vi "IMAQ-MWT DUAL DMD Intensity Calibration (HOST).vi"() -> ()   [LabVIEW 2017]
uses:
  Modules/Common/Controls (HOST)/Image Size.ctl
  Modules/Common/Controls (HOST)/REF.ctl
  Modules/Common/Controls (HOST)/Image Queue Bundle.ctl
  Modules/Common/Controls (HOST)/Data to Disk Bundle.ctl
  Modules/Common/Controls (HOST)/File Name Prefix.ctl
  Modules/Common/Controls (HOST)/FPGA REF (MWT).ctl
  Modules/Common/Controls (HOST)/Main States.ctl
  Modules/Common/Controls (HOST)/IMAQ Parameters.ctl
  Modules/Common/Controls (HOST)/File REF.ctl
  <vilib>/vision/Avi.llb/IMAQ AVI2 Refnum.ctl
  Modules/Common/Controls (HOST)/Experiment Mode.ctl
  <vilib>/Utility/error.llb/Error Cluster From Error Code.vi
  <vilib>/rvi/errors/niLvFpgaAdjustHostInterfaceError.vi
  <vilib>/FPGAPlugInAG/Dynamic/niLvFpga_Close_Dynamic.vi
  <vilib>/Utility/file.llb/Read Delimited Spreadsheet (DBL).vi
  <vilib>/Utility/file.llb/Write Delimited Spreadsheet (DBL).vi
  <vilib>/rvi/interface/nirviReadWriteControl/nirviReadWriteControl.xnode
  <vilib>/rvi/interface/nirviCloseFPGA/nirviCloseFPGA.xnode
  NiFpgaLv.dll
  <vilib>/rvi/interface/Simulation/niFpgaSimulationCallBeginRW.vi
panel:
  in  "Rows Complete":i32
  in  "Int Coeff":bool
  in  "Intensity (mW/cm2)":dbl[][](array[numeric])
  in  "Save Int":bool
  in  "Measured Intensity (uW/cm2)":dbl format="%.2f"
  in  "Current Measurement Spot":cluster{"Rows":u32, "Columns":u32}={"Rows"=1, "Columns"=1} {"Columns" min=1 step=1; "Rows" min=1 step=1}
  out "Total Number of Calibration Points":u32
  in  "Number of Calibration Points":cluster{"Rows":u32, "Columns":u32}={"Rows"=4, "Columns"=4}
  in  "Image Size":T1={"Height"=3072, "Width"=3200}
  out "Frame Rate":u32
  out "Frame #":u32
  in  "Stop Button":bool
  in  "Go":bool
  in  "Height":i32=100
  in  "Width":i32=100
  in  "Y":i32=334
  in  "X":i32=462
  out "Exp. Status":string="Camera Connected"
  out "REF":T2
  out "Command Q":refnum<queue>
  out "Display":T5(plugin-control)
  out "Stopped?":bool
  # "DUAL DMD Intensity Calibration"
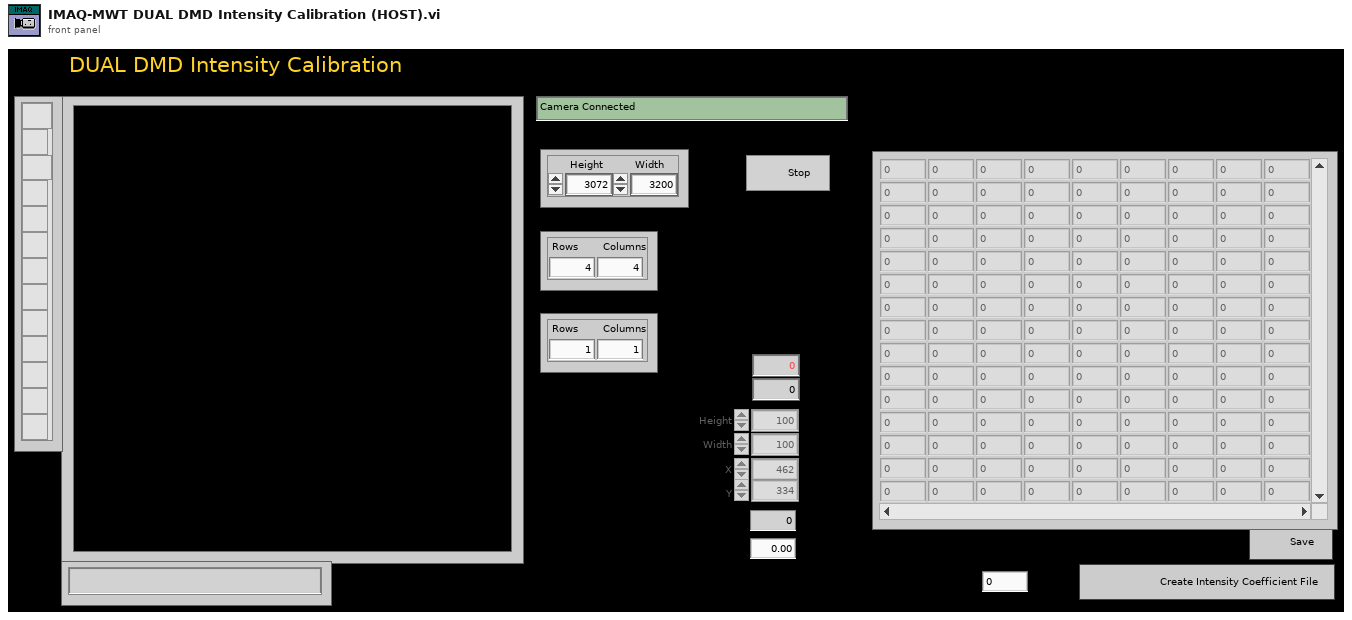
[diagram p1: front panel]
types:
  T1 = typedef "Image Size.ctl" = cluster{"Height":u16, "Width":u16}
  T2 = typedef "REF.ctl" = cluster{"Queue REF":T3, "FPGA REF (MWT)":T4}
  T3 = typedef "Image Queue Bundle.ctl" = cluster{"Disk Image":refnum<queue>, "Image Blocks":refnum<queue>, "Display Image":refnum<queue>, "BG Image":refnum<queue>, "Tag Image":refnum<queue>, "DLL Input":refnum<queue>, "DMD Input":refnum<queue>, "GALVO Input":refnum<queue>}
  T4 = typedef "FPGA REF (MWT).ctl" = refnum<k20>
  T5 = typedef "IMAQ Image.ctl" = refnum<image>
  T6 = enum8{"Enabled", "Disabled", "Disabled and Grayed Out"}
  T7 = typedef "Main States.ctl" = enum16{"Open FPGA", "Initialize", "Preview", "Acquire Images", "STOP"}
  T8 = typedef "Experiment Mode.ctl" = enum16{"Live", "Replay"}
  T9 = typedef "IMAQ Parameters.ctl" = cluster{"File REF":T10, "Frame Data":cluster{"Width":u32, "Height":u32, "Frames Per Second":u32, "Codec":string}, "File Type":string, "Experiment Mode":T8, "Movie File Path":path}
  T10 = typedef "File REF.ctl" = cluster{"AVI REF":T11, "DBDE REF":refnum<file>}
  T11 = typedef "IMAQ AVI2 Refnum.ctl" = refnum<k20>
  T12 = typedef "Data to Disk Bundle.ctl" = cluster{"Frame Number":u64, "Time Stamp (us)":u64, "Image Data":u64[], "Contour":u32[], "Raw Image REF":refnum<data-value>, "Block Image REF":refnum<data-value>, "Block Box":u64[], "SPINE":u32[], "HT Angle":u64[], "Block Position":u64[], "SPINE Count":u32[], "Contour Count":u32[], "SPINE DIR":u8[]}
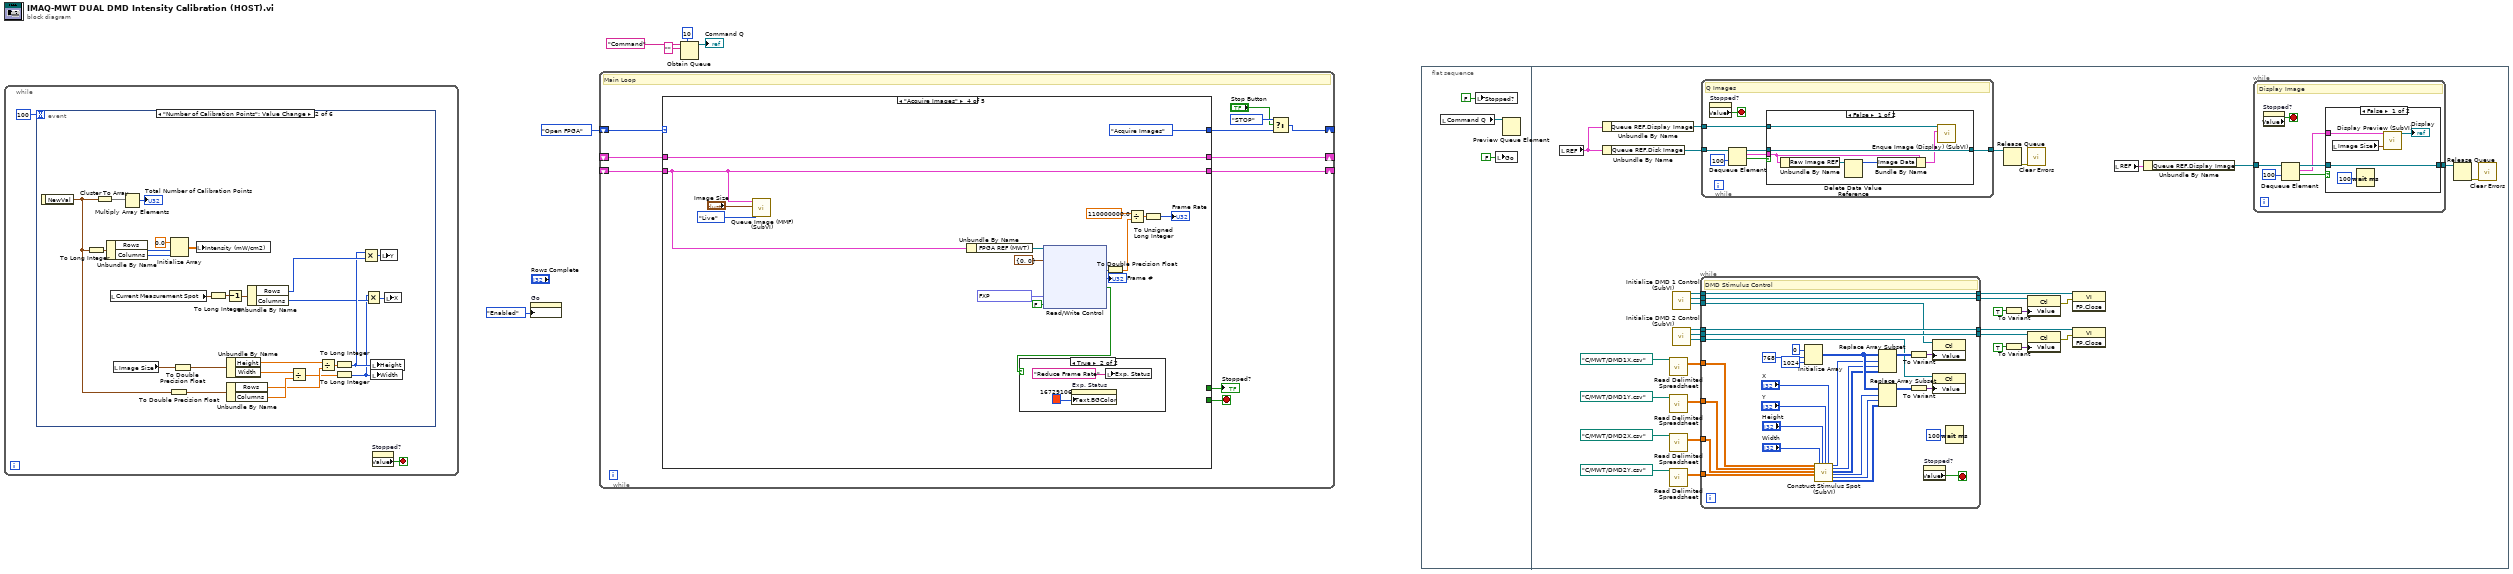
[diagram p0: block diagram]
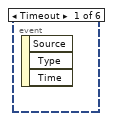
[diagram p2: hidden frame]
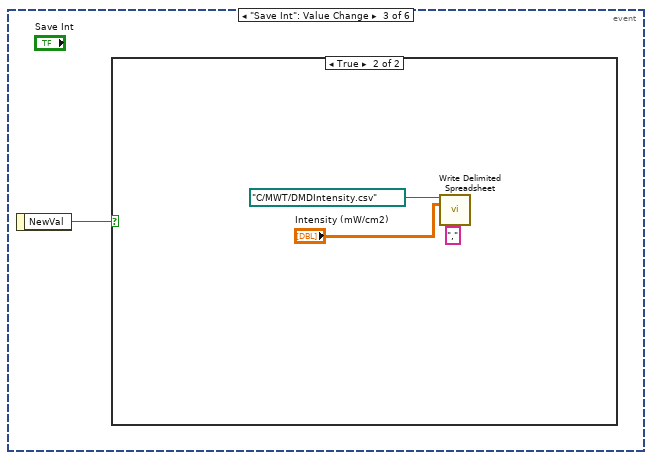
[diagram p3: hidden frame]
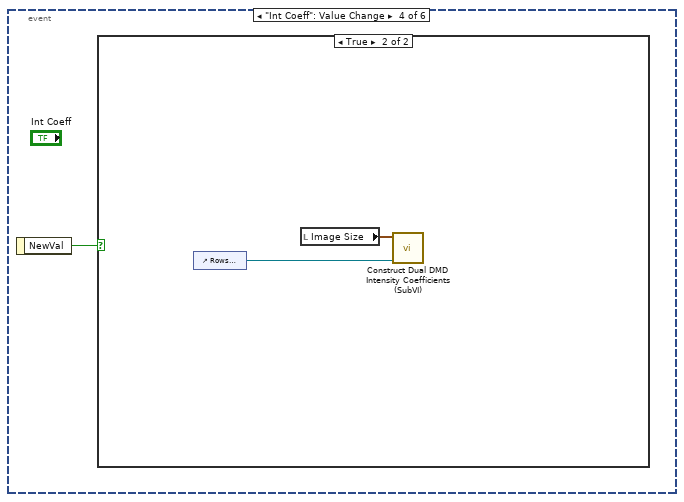
[diagram p5: hidden frame]
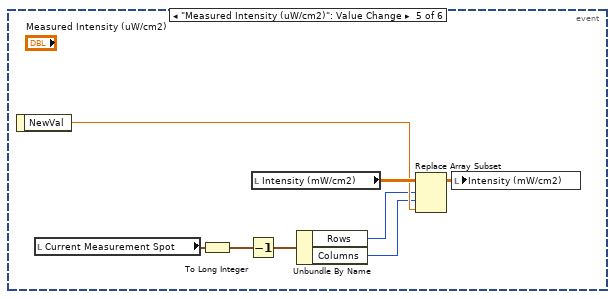
[diagram p7: hidden frame]
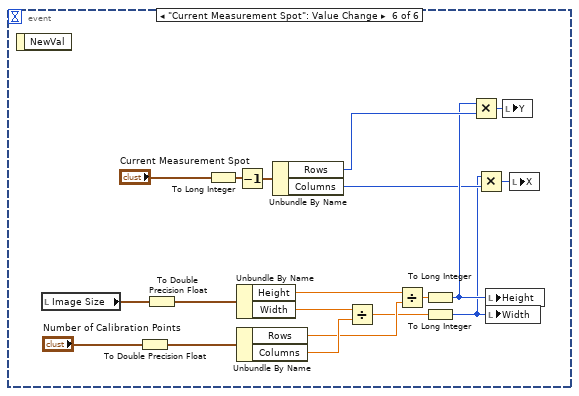
[diagram p8: hidden frame]
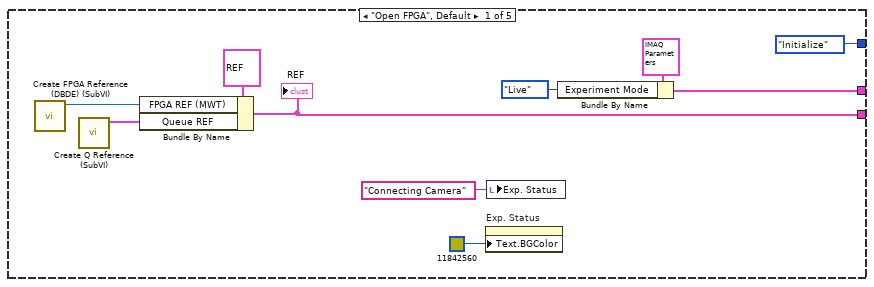
[diagram p11: hidden frame]
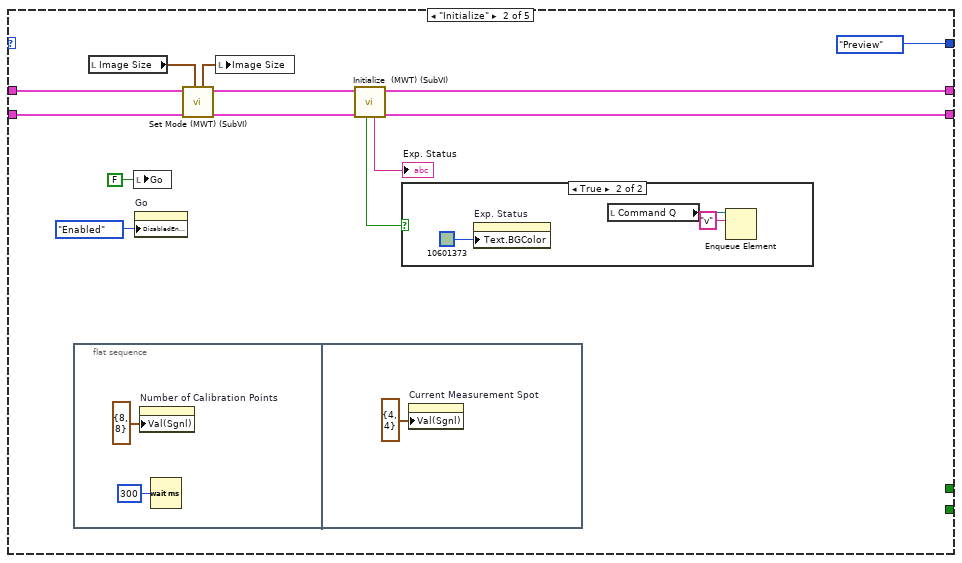
[diagram p12: hidden frame]
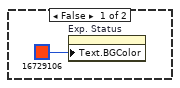
[diagram p13: hidden frame]
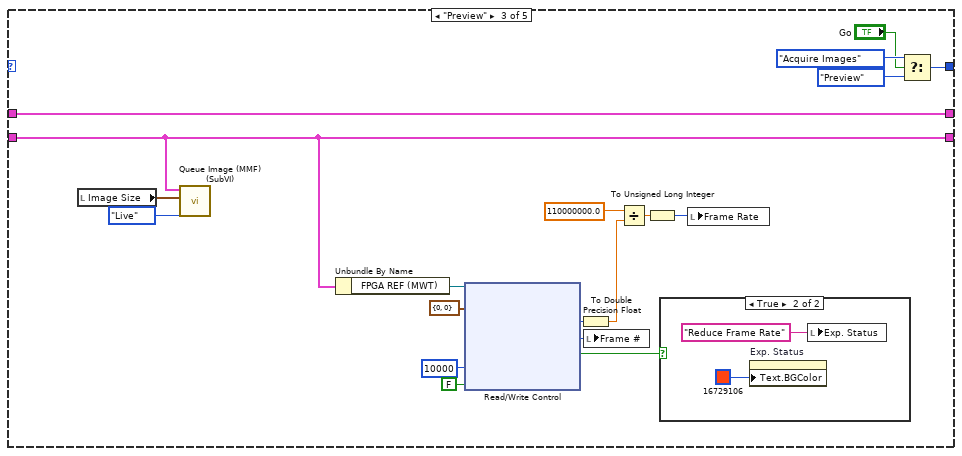
[diagram p14: hidden frame]
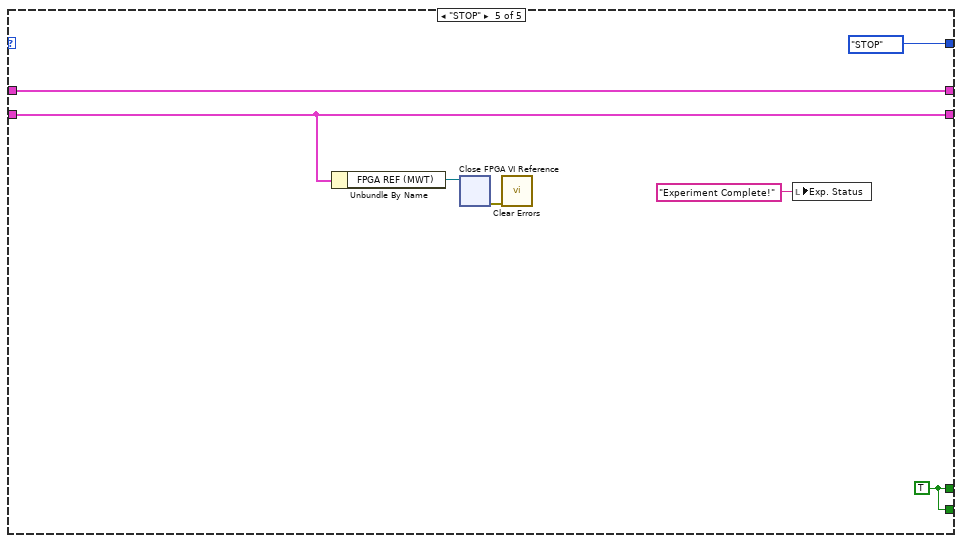
[diagram p17: hidden frame]
diagram:
  n1 = while {
    stop <- w8 stop-if-true
    n2 = event shown="[1] \"Number of Calibration Points\": Value Change" {
      selector: _ -> [_ _ _ _ _ _]
      dyn-events: _ -> [_ _ _ _ _ _]
      timeout: 100 -> [_ _ _ _ _ _]
      event Timeout {
        n3 = event-data() -> ()  [unwired: 1 in, 3 out]
      }
      event "Number of Calibration Points": Value Change {
        n4 = event-data() -> ("NewVal"=w9:cluster{"Rows":u32, "Columns":u32})  [unwired: 1 in]
        n5 = To Long Integer(number=w9) -> (32bit integer=w29:cluster{"Rows":i32, "Columns":i32})
        n6 = Cluster To Array(cluster=w9) -> (array=w33:u32[])
        n7 = Unbundle By Name(w29) -> ("Rows"=w32:i32, "Columns"=w31:i32)
        n8 = local read "Current Measurement Spot"() -> (w27:cluster{"Rows":u32, "Columns":u32})
        n9 = local read "Image Size"() -> (w26:T1)
        n10 = Multiply Array Elements(1:w33) -> (0:→"Total Number of Calibration Points":u32)
        n11 = To Double Precision Float(number=w9) -> (double precision float=w24:cluster{"Rows":dbl, "Columns":dbl})
        n12 = Initialize Array(0.0 ("element"), w32, w31) -> (w28:dbl[][])
        n13 = To Double Precision Float(number=w26) -> (double precision float=w25:cluster{"Height":dbl, "Width":dbl})
        n14 = local write "Intensity (mW/cm2)"(w28) -> ()
        n15 = To Long Integer(number=w27) -> (32bit integer=w14:cluster{"Rows":i32, "Columns":i32})
        n16 = Decrement(x=w14) -> (x-1=w17:cluster{"Rows":i32, "Columns":i32})
        n17 = Unbundle By Name(w25) -> ("Height"=w23:dbl, "Width"=w22:dbl)
        n18 = Unbundle By Name(w24) -> ("Rows"=w20:dbl, "Columns"=w21:dbl)
        n19 = Unbundle By Name(w17) -> ("Rows"=w16:i32, "Columns"=w11:i32)
        n20 = Divide(x=w22, y=w21) -> (x/y=w19:dbl)
        n21 = Divide(x=w23, y=w20) -> (x/y=w18:dbl)
        n22 = To Long Integer(number=w18) -> (32bit integer=w13:i32)
        n23 = To Long Integer(number=w19) -> (32bit integer=w10:i32)
        n24 = Multiply(x=w13, y=w16) -> (x*y=w15:i32)
        n25 = Multiply(x=w10, y=w11) -> (x*y=w12:i32)
        n26 = local write "Height"(w13) -> ()
        n27 = local write "Width"(w10) -> ()
        n28 = local write "Y"(w15) -> ()
        n29 = local write "X"(w12) -> ()
      }
      event "Save Int": Value Change {
        n30 = event-data() -> ("NewVal"=w35:bool)  [unwired: 1 in]
        n31 = case shown="True" w35 {
          frame False {
          }
          frame True {
            n32 = call-poly <vilib>:"Write Delimited Spreadsheet.vi"("file path (dialog if empty)"=path "C:/MWT/DMDIntensity.csv", "2D data"="Intensity (mW/cm2)", "delimiter (\\t)"="," ("delimiter (\\t)")) -> ()  [unwired: 11 in, 2 out]
          }
        }
      }
      event "Int Coeff": Value Change {
        n33 = event-data() -> ("NewVal"=w39:bool)  [unwired: 1 in]
        n34 = case shown="True" w39 {
          frame False {
          }
          frame True {
            n35 = control-ref of="Rows Complete"() -> (w40:refnum<vi>)
            n36 = local read "Image Size"() -> (w41:T1)
            n37 = call "Construct Dual DMD Intensity Coefficients (SubVI).vi"("Number of Rows Processed"=w40, "Image Size in"=w41) -> ()  [unwired: 10 in]
          }
        }
      }
      event "Measured Intensity (uW/cm2)": Value Change {
        n38 = event-data() -> ("NewVal"=w48:dbl)  [unwired: 1 in]
        n39 = local read "Current Measurement Spot"() -> (w47:cluster{"Rows":u32, "Columns":u32})
        n40 = To Long Integer(number=w47) -> (32bit integer=w44:cluster{"Rows":i32, "Columns":i32})
        n41 = Decrement(x=w44) -> (x-1=w42:cluster{"Rows":i32, "Columns":i32})
        n42 = local read "Intensity (mW/cm2)"() -> (w49:dbl[][])
        n43 = Unbundle By Name(w42) -> ("Rows"=w46:i32, "Columns"=w45:i32)
        n44 = Replace Array Subset(array=w49, new element=w48, index (row)=w46, index (col)=w45) -> (w43:dbl[][])
        n45 = local write "Intensity (mW/cm2)"(w43) -> ()
      }
      event "Current Measurement Spot": Value Change {
        n46 = event-data() -> ()  [unwired: 1 in, 1 out]
        n47 = local read "Image Size"() -> (w68:T1)
        n48 = To Double Precision Float(number="Number of Calibration Points") -> (double precision float=w65:cluster{"Rows":dbl, "Columns":dbl})
        n49 = To Double Precision Float(number=w68) -> (double precision float=w66:cluster{"Height":dbl, "Width":dbl})
        n50 = To Long Integer(number="Current Measurement Spot") -> (32bit integer=w55:cluster{"Rows":i32, "Columns":i32})
        n51 = Decrement(x=w55) -> (x-1=w58:cluster{"Rows":i32, "Columns":i32})
        n52 = Unbundle By Name(w66) -> ("Height"=w64:dbl, "Width"=w63:dbl)
        n53 = Unbundle By Name(w65) -> ("Rows"=w61:dbl, "Columns"=w62:dbl)
        n54 = Unbundle By Name(w58) -> ("Rows"=w57:i32, "Columns"=w52:i32)
        n55 = Divide(x=w63, y=w62) -> (x/y=w60:dbl)
        n56 = Divide(x=w64, y=w61) -> (x/y=w59:dbl)
        n57 = To Long Integer(number=w59) -> (32bit integer=w54:i32)
        n58 = To Long Integer(number=w60) -> (32bit integer=w51:i32)
        n59 = Multiply(x=w54, y=w57) -> (x*y=w56:i32)
        n60 = Multiply(x=w51, y=w52) -> (x*y=w53:i32)
        n61 = local write "Height"(w54) -> ()
        n62 = local write "Width"(w51) -> ()
        n63 = local write "Y"(w56) -> ()
        n64 = local write "X"(w53) -> ()
      }
    }
    n65 = property on="Stopped?" class="Bool (strict)"() -> ("Value"=w8:bool)  [unwired: 2 in, 2 out]
  }
  n66 = property on="Go" class="Bool (strict)"("DisabledEnum"=T6."Enabled" ("Disabled")) -> ()  [unwired: 2 in, 2 out]
  n67 = while {
    shift-right: [w78] -> _
    shift-left: _ -> [w77]
    shift-right: [w69] -> _
    shift-left: Main_States."Open FPGA" -> [w79]
    shift-right: [w71] -> _
    shift-left: _ -> [w70]
    stop <- w75 stop-if-true
    # "Main Loop"
    n68 = case shown="\"Acquire Images\"" w79 {
      tunnel: [w86 w90 w114 w136 w152] -> w78
      tunnel: w77 -> [_ w91 w114 w136 w152]
      tunnel: [Main_States."Initialize" Main_States."Preview" w127 Main_States."Acquire Images" Main_States."STOP"] -> w76
      tunnel: [_ _ _ _ w154] -> w75
      tunnel: [_ _ _ _ w154] -> w74
      tunnel: [w81 w95 w120 w137 w151] -> w71
      tunnel: w70 -> [_ w101 w120 w137 w151]
      frame "Open FPGA", Default {
        n69 = call "Create FPGA Reference (DBDE) (SubVI).vi"() -> ("FPGA REF (MWT)"=w88:T4)  [unwired: 11 in]
        n70 = call "Create Q Reference (SubVI).vi"() -> ("Image Queue"=w87:T3)  [unwired: 11 in]
        n71 = Bundle By Name(cluster=T2 {"Queue REF"={"Disk Image"=refnum, "Image Blocks"=refnum, "Display Image"=refnum, "BG Image"=refnum, "Tag Image"=refnum, "DLL Input"=refnum, "DMD Input"=refnum, "GALVO Input"=refnum}, "FPGA REF (MWT)"=refnum}, "FPGA REF (MWT)"=w88, "Queue REF"=w87) -> (w86:T2)
        "REF" <- w86
        n72 = property on="Exp. Status" class="Str"("Text.BGColor"=u32 11842560) -> ()  [unwired: 2 in, 2 out]
        n73 = local write "Exp. Status"("Connecting Camera" ("Exp. Status")) -> ()
        n74 = Bundle By Name(cluster=T9 {"File REF"={"AVI REF"=refnum, "DBDE REF"=refnum}, "Frame Data"={"Width"=0, "Height"=0, "Frames Per Second"=0, "Codec"=""}, "File Type"="", "Experiment Mode"=enum."Live", "Movie File Path"=path "D:/Movies Formatted on November 5th 2015/Clip (2) Formatted.raw"} ("Movie File Property"), "Experiment Mode"=Experiment_Mode."Live") -> (w81:T9)
      }
      frame "Initialize" {
        n75 = flat-sequence {
          frame #0 {
            n76 = property on="Number of Calibration Points" class="Clust (strict)"("Val(Sgnl)"=cluster{"Rows":u32, "Columns":u32} {"Rows"=8, "Columns"=8} ("Value (Signaling)")) -> ()  [unwired: 2 in, 2 out]
            n77 = Wait (ms)(milliseconds to wait=u32 300) -> ()  [unwired: 1 out]
          }
          frame #1 {
            n78 = property on="Current Measurement Spot" class="Clust (strict)"("Val(Sgnl)"=cluster{"Rows":u32, "Columns":u32} {"Rows"=4, "Columns"=4} ("Value (Signaling)")) -> ()  [unwired: 2 in, 2 out]
          }
        }
        n79 = local read "Image Size"() -> (w93:T1)
        n80 = local write "Go"(FALSE ("Go")) -> ()
        n81 = property on="Go" class="Bool (strict)"("DisabledEnum"=T6."Enabled" ("Disabled")) -> ()  [unwired: 2 in, 2 out]
        n82 = call "Set Mode (MWT) (SubVI).vi"("Image Size In"=w93, "REF IN"=w91, "Parameters In"=w101) -> ("REF OUT"=w94:T2, "Parameters Out"=w96:T9, "Image Size Out"=w92:T1)  [unwired: 6 in]
        n83 = local write "Image Size"(w92) -> ()
        n84 = call "Initialize  (MWT) (SubVI).vi"("REF IN"=w94, "Parameters In"=w96) -> ("REF OUT"=w90:T2, "Parameters Out"=w95:T9, "Exp. Status"=→"Exp. Status":string, "OK?"=w98:bool)  [unwired: 6 in]
        n85 = case shown="True" w98 {
          frame False {
            n86 = property on="Exp. Status" class="Str"("Text.BGColor"=u32 16729106) -> ()  [unwired: 2 in, 2 out]
          }
          frame True {
            n87 = property on="Exp. Status" class="Str"("Text.BGColor"=u32 10601373) -> ()  [unwired: 2 in, 2 out]
            n88 = local read "Command Q"() -> (w108:refnum<queue>)
            n89 = Enqueue Element(queue=w108, element="v") -> ()  [unwired: 2 in, 3 out]
          }
        }
      }
      frame "Preview" {
        n90 = local read "Image Size"() -> (w117:T1)
        n91 = call "Queue Image (MMF) (SubVI).vi"("Experiment Mode"=Experiment_Mode."Live", "Image Size"=w117, "Data Bundle"=w114) -> ()  [unwired: 9 in]
        n92 = Unbundle By Name(w114) -> ("FPGA REF (MWT)"=w123:T4)
        n93 = xnode "Read/Write Control"("FPGA VI Reference In"=w123, "Pixel Intensity"=cluster{"Low":u8, "High":u8} {"Low"=0, "High"=0}, "Clock Cycles Limit"=u32 10000, "Swap Bytes"=FALSE) -> ("Frame Interval"=w125:u32, "Frame #"=w116:u32, "DMA Timeout"=w115:bool)  [unwired: 1 in, 2 out]
        n94 = To Double Precision Float(number=w125) -> (double precision float=w124:dbl)
        n95 = local write "Frame #"(w116) -> ()
        n96 = Divide(x=110000000.0 ("y"), y=w124) -> (x/y=w121:dbl)
        n97 = To Unsigned Long Integer(number=w121) -> (unsigned 32bit integer=w119:u32)
        n98 = case shown="True" w115 {
          frame False {
          }
          frame True {
            n99 = property on="Exp. Status" class="Str"("Text.BGColor"=u32 16729106) -> ()  [unwired: 2 in, 2 out]
            n100 = local write "Exp. Status"("Reduce Frame Rate" ("Exp. Status")) -> ()
          }
        }
        n101 = local write "Frame Rate"(w119) -> ()
        n102 = Select(t=Main_States."Acquire Images", s="Go", f=Main_States."Preview") -> (s? t:f=w127:T7)
      }
      frame "Acquire Images" {
        n103 = call "Queue Image (MMF) (SubVI).vi"("Experiment Mode"=Experiment_Mode."Live", "Image Size"="Image Size", "Data Bundle"=w136) -> ()  [unwired: 9 in]
        n104 = Unbundle By Name(w136) -> ("FPGA REF (MWT)"=w143:T4)
        n105 = xnode "Read/Write Control"("FPGA VI Reference In"=w143, "Pixel Intensity"=cluster{"Low":u8, "High":u8} {"Low"=0, "High"=0}, "Significant Angle"=fxp<+,16,3> 0.0699462890625, "Swap Bytes"=FALSE) -> ("Frame Interval"=w145:u32, "Frame #"=→"Frame #":u32, "DMA Timeout"=w138:bool)  [unwired: 1 in, 2 out]
        n106 = case shown="True" w138 {
          frame False {
          }
          frame True {
            n107 = property on="Exp. Status" class="Str"("Text.BGColor"=u32 16729106) -> ()  [unwired: 2 in, 2 out]
            n108 = local write "Exp. Status"("Reduce Frame Rate" ("Exp. Status")) -> ()
          }
        }
        n109 = To Double Precision Float(number=w145) -> (double precision float=w144:dbl)
        n110 = Divide(x=110000000.0 ("y"), y=w144) -> (x/y=w140:dbl)
        n111 = To Unsigned Long Integer(number=w140) -> (unsigned 32bit integer=→"Frame Rate":u32)
      }
      frame "STOP" {
        w154 = TRUE
        n112 = Unbundle By Name(w152) -> ("FPGA REF (MWT)"=w153:T4)
        n113 = xnode "Close FPGA VI Reference"("FPGA VI Reference In"=w153) -> ("error out"=w149:errorcluster)  [unwired: 1 in]
        n114 = call <vilib>:"Clear Errors.vi"("error in (no error)"=w149) -> ()  [unwired: 5 in, 2 out]
        n115 = local write "Exp. Status"("Experiment Complete!" ("Exp. Status")) -> ()
      }
    }
    "Stopped?" <- w74
    n116 = Select(t=Main_States."STOP", s="Stop Button", f=w76) -> (s? t:f=w69:T7)
  }
  n117 = Obtain Queue(max queue size (-1, unlimited)=10, name (unnamed)="Command", element data type="" ("name (unnamed)")) -> (queue out=→"Command Q":refnum<queue>)  [unwired: 2 in, 2 out]
  n118 = flat-sequence {
    frame #0 {
      n119 = local read "Command Q"() -> (w158:refnum<queue>)
      n120 = local write "Stopped?"(FALSE ("Stopped?")) -> ()
      n121 = local write "Go"(FALSE ("Go")) -> ()
      n122 = Preview Queue Element(queue=w158) -> ()  [unwired: 2 in, 4 out]
    }
    frame #1 {
      n123 = local read "REF"() -> (w185:T2)
      n124 = Unbundle By Name(w185) -> ("Queue REF.Display Image"=w186:refnum<queue>)
      n125 = Unbundle By Name(w185) -> ("Queue REF.Disk Image"=w187:refnum<queue>)
      n126 = call-poly <vilib>:"Read Delimited Spreadsheet.vi"("file path (dialog if empty)"=path "C:/MWT/DMD1X.csv") -> ("all rows"=w162:dbl[][])  [unwired: 9 in, 5 out]
      n127 = call-poly <vilib>:"Read Delimited Spreadsheet.vi"("file path (dialog if empty)"=path "C:/MWT/DMD1Y.csv") -> ("all rows"=w161:dbl[][])  [unwired: 9 in, 5 out]
      n128 = call-poly <vilib>:"Read Delimited Spreadsheet.vi"("file path (dialog if empty)"=path "C:/MWT/DMD2X.csv") -> ("all rows"=w160:dbl[][])  [unwired: 9 in, 5 out]
      n129 = call-poly <vilib>:"Read Delimited Spreadsheet.vi"("file path (dialog if empty)"=path "C:/MWT/DMD2Y.csv") -> ("all rows"=w159:dbl[][])  [unwired: 9 in, 5 out]
      n130 = call "Initialize DMD 1 Control (SubVI).vi"() -> ("DMD IMG REF"=w168:refnum<vi>, "STOP REF"=w169:refnum<vi>, "DMD VI REF"=w170:refnum<vi>)  [unwired: 9 in]
      n131 = call "Initialize DMD 2 Control (SubVI).vi"() -> ("DMD IMG REF"=w175:refnum<vi>, "STOP REF"=w181:refnum<vi>, "DMD VI REF"=w182:refnum<vi>)  [unwired: 9 in]
      n132 = while {
        tunnel: w182 -> [w219]
        tunnel: w181 -> [w220]
        tunnel: [w220] -> w179
        tunnel: [w219] -> w176
        tunnel: w175 -> [w206]
        tunnel: w170 -> [w218]
        tunnel: w169 -> [w217]
        tunnel: [w217] -> w172
        tunnel: [w218] -> w174
        tunnel: w168 -> [w207]
        tunnel: w162 -> [w205]
        tunnel: w161 -> [w204]
        tunnel: w160 -> [w203]
        tunnel: w159 -> [w202]
        stop <- w221 stop-if-true
        # "DMD Stimulus Control"
        n133 = Initialize Array(u8 0 ("element"), 768 ("dimension size"), 1024 ("dimension size")) -> (w210:u8[][])
        n134 = call "Construct Stimulus Spot (SubVI).vi"("DMD1X Array"=w205, "DMD1Y Array"=w204, "DMD2X Array"=w203, "DMD2Y Array"=w202, "Width"="Width", "Height"="Height", "Y"="Y", "X"="X") -> ("DMD1Y"=w197:i32, "DMD1X"=w196:i32, "DMD1 Array"=w195:u8[][], "DMD2Y"=w194:i32, "DMD2X"=w193:i32, "DMD2 Array"=w192:u8[][])  [unwired: 6 in]
        n135 = Replace Array Subset(array=w210, new element=w195, index (row)=w197, index (col)=w196) -> (w216:u8[][])
        n136 = Replace Array Subset(array=w210, new element=w192, index (row)=w194, index (col)=w193) -> (w208:u8[][])
        n137 = To Variant(anything=w216) -> (Variant=w215:variant)
        n138 = To Variant(anything=w208) -> (Variant=w209:variant)
        n139 = property on="Stopped?" class="Bool (strict)"() -> ("Value"=w221:bool)  [unwired: 2 in, 2 out]
        n140 = property class="Ctl"(reference=w207, "Value"=w215) -> ()  [unwired: 1 in, 2 out]
        n141 = property class="Ctl"(reference=w206, "Value"=w209) -> ()  [unwired: 1 in, 2 out]
        n142 = Wait (ms)(milliseconds to wait=u32 100) -> ()  [unwired: 1 out]
      }
      n143 = while {
        tunnel: [w228] -> w188
        tunnel: w187 -> [w222]
        tunnel: w186 -> [w227]
        stop <- w223 stop-if-true
        # "Q Images"
        n144 = property on="Stopped?" class="Bool (strict)"() -> ("Value"=w223:bool)  [unwired: 2 in, 2 out]
        n145 = Dequeue Element(queue=w222, timeout in ms (-1)=100) -> (queue out=w225:refnum<queue>, element=w226:T12, timed out?=w224:bool)  [unwired: 1 in, 1 out]
        n146 = case shown="False" w224 {
          tunnel: w225 -> [w235 w236]
          tunnel: [w235 w236] -> w228
          tunnel: w227 -> [w234 _]
          tunnel: w226 -> [w232 _]
          frame False {
            n147 = Unbundle By Name(w232) -> ("Raw Image REF"=w233:refnum<data-value>)
            n148 = Delete Data Value Reference(data value reference=w233) -> (data value=w231:u64[])  [unwired: 1 in, 1 out]
            n149 = Bundle By Name(cluster=w232, "Image Data"=w231) -> (w230:T12)
            n150 = call "Enque Image (Display) (SubVI).vi"("Data Bundle"=w230, "Display Image REF"=w234) -> ()  [unwired: 10 in]
          }
          frame True {
          }
        }
      }
      n151 = Release Queue(queue=w188) -> (error out=w183:errorcluster)  [unwired: 2 in, 2 out]
      n152 = To Variant(anything=TRUE ("Wait Until Done")) -> (Variant=w171:variant)
      n153 = To Variant(anything=TRUE ("Wait Until Done")) -> (Variant=w180:variant)
      n154 = call <vilib>:"Clear Errors.vi"("error in (no error)"=w183) -> ()  [unwired: 5 in, 2 out]
      n155 = property class="Ctl"(reference=w172, "Value"=w171) -> (error out=w173:errorcluster)  [unwired: 1 in, 1 out]
      n156 = property class="Ctl"(reference=w179, "Value"=w180) -> (error out=w177:errorcluster)  [unwired: 1 in, 1 out]
      n157 = invoke class="VI" method="FP.Close"(reference=w174, error in=w173) -> ()  [unwired: 1 in, 3 out]
      n158 = invoke class="VI" method="FP.Close"(reference=w176, error in=w177) -> ()  [unwired: 1 in, 3 out]
      n159 = local read "REF"() -> (w190:T2)
      n160 = Unbundle By Name(w190) -> ("Queue REF.Display Image"=w189:refnum<queue>)
      n161 = while {
        tunnel: [w240] -> w191
        tunnel: w189 -> [w239]
        stop <- w237 stop-if-true
        # "Display Image"
        n162 = property on="Stopped?" class="Bool (strict)"() -> ("Value"=w237:bool)  [unwired: 2 in, 2 out]
        n163 = Dequeue Element(queue=w239, timeout in ms (-1)=100) -> (queue out=w241:refnum<queue>, element=w238:T12, timed out?=w242:bool)  [unwired: 1 in, 1 out]
        n164 = case shown="False" w242 {
          tunnel: w241 -> [w248 w249]
          tunnel: [w248 w249] -> w240
          tunnel: w238 -> [w247 _]
          frame False {
            n165 = local read "Image Size"() -> (w245:T1)
            n166 = Wait (ms)(milliseconds to wait=u32 100) -> ()  [unwired: 1 out]
            n167 = call "Display Preview (SubVI).vi"("Display Data"=w247, "Image Size"=w245) -> ("Image Out"=→"Display":T5)  [unwired: 17 in]
          }
          frame True {
          }
        }
      }
      n168 = Release Queue(queue=w191) -> (error out=w184:errorcluster)  [unwired: 2 in, 2 out]
      n169 = call <vilib>:"Clear Errors.vi"("error in (no error)"=w184) -> ()  [unwired: 5 in, 2 out]
    }
  }
